vi "extractObjectPrivateDataValues.vi"(7 "error in (no error)":errorcluster, 8 "classPrivateDataDefaults":variant[](array[variant]), 9 "Object in":refnum<class>) -> (0 "error out":errorcluster, 2 "objectPrivateData":variant[](array[variant]))   [LabVIEW 2020, in "openg_variant.lvlib" / "Reflection.lvclass"]
doc: "Returns object Private Data values for the complete class hierarchy.\nClass Private Data defaults must be passed as an array of Variants where each element is a cluster of class private data with element 0 being the current class and the last element is the top ancestor class.\n\nGCraftsman JSON Object Serialization Toolkit\nwww.GCraftsman.com\nCopyright (c) 2017, GCraftsman"
uses:
  Reflection.lvclass
  Reflection.lvclass/Reflection.ctl
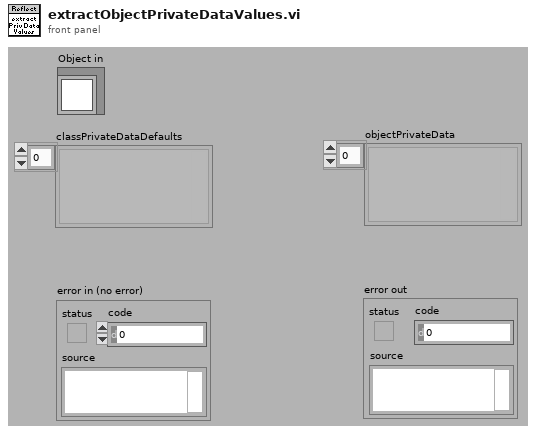
[diagram p1: front panel]
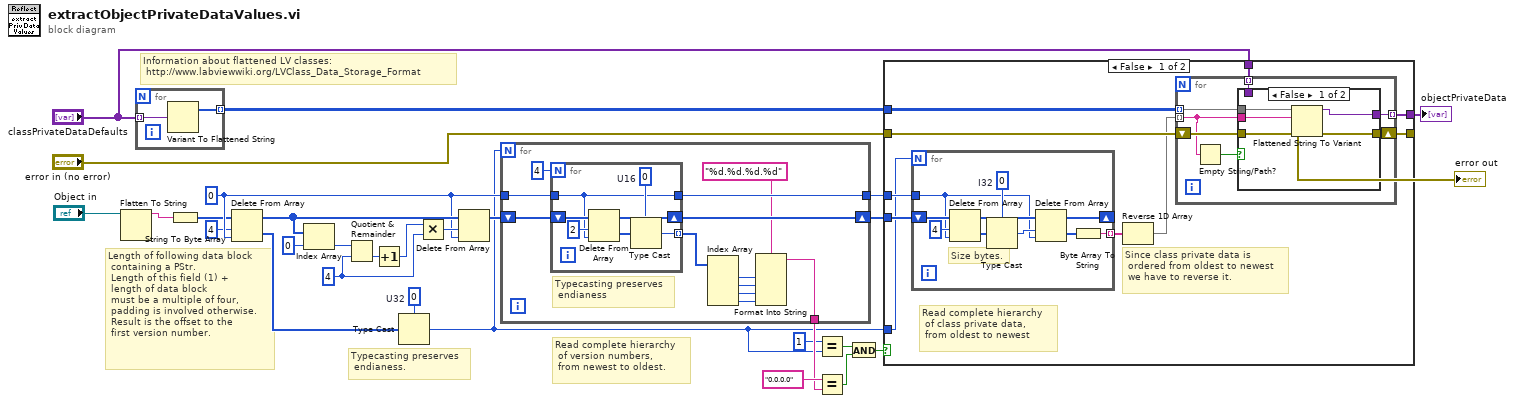
[diagram p0: block diagram]
diagram:
  w4 = u32 0  # U32
  w8 = u8 4 ("y")
  w19 = 0 ("index")
  # "Read complete hierarchy\n of version numbers,\n from newest to oldest."
  # "Information about flattened LV classes:\n http://www.labviewwiki.org/LVClass_Data_Storage_Format"
  # "Typecasting preserves\n endianess."
  # "Length of following data block\n containing a PStr.\n Length of this field (1) +\n length of data block\n must be a multiple of four,\n padding is involved otherwise.\n Result is the offset to the\n first version number."
  n1 = Flatten To String(anything="Object in") -> (data string=w1:string)  [unwired: 3 in, 2 out]
  n2 = for {
    tunnel: [w31] -> w14 mode=indexing
    tunnel: "classPrivateDataDefaults" -> [w30] mode=indexing
    n3 = Variant To Flattened String(Variant=w30) -> (1:w31:i16[])  [unwired: 1 out]
  }
  n4 = String To Byte Array(string=w1) -> (unsigned byte array=w16:u8[])
  n5 = Delete From Array(array=w16, length=4 ("offset (0)"), index=w19) -> (deleted portion=w6:u8[], array with subset deleted=w22:u8[])
  n6 = Index Array(array=w22, index=0) -> (element=w11:u8)
  n7 = Quotient & Remainder(x=w11, y=w8) -> (floor(x/y)=w10:u8)  [unwired: 1 out]
  n8 = Increment(x=w10) -> (x+1=w9:u8)
  n9 = Type Cast(type=w4, x=w6) -> (*(type *) &x=w5:u32)
  n10 = Multiply(x=w9, y=w8) -> (x*y=w21:u8)
  n11 = Delete From Array(array=w22, length=w21, index=w19) -> (array with subset deleted=w17:u8[])  [unwired: 1 out]
  n12 = for {
    N: w5 -> [_]
    shift-right: [w42] -> w18
    shift-left: w17 -> [w43]
    tunnel: w19 -> [w41]
    tunnel: [w39] -> w20
    tunnel: [w40] -> w24
    # "Typecasting preserves\n endianess"
    n13 = for {
      N: 4 -> [_]
      shift-right: [w48] -> w42
      shift-left: w43 -> [w50]
      tunnel: w41 -> [w44]
      tunnel: [w45] -> w36 mode=indexing
      tunnel: [w44] -> w39
      w46 = u16 0  # U16
      n14 = Delete From Array(array=w50, length=2, index=w44) -> (deleted portion=w47:u8[], array with subset deleted=w48:u8[])
      n15 = Type Cast(type=w46, x=w47) -> (*(type *) &x=w45:u16)
    }
    n16 = Index Array(array=w36) -> (element #1=w35:u16, element #2=w34:u16, element #3=w33:u16, element #4=w32:u16)  [unwired: 4 in]
    n17 = Format Into String(format string="%d.%d.%d.%d", w35, w34, w33, w32) -> (resulting string=w40:string)  [unwired: 2 in, 1 out]
  }
  n18 = Equal?(x=u32 1, y=w5) -> (x = y?=w26:bool)
  n19 = Equal?(x="0.0.0.0", y=w24) -> (x = y?=w27:bool)
  n20 = And(x=w26, y=w27) -> (x .and. y?=w28:bool)
  n21 = case shown="False" w28 {
    tunnel: w14 -> [w60 _]
    tunnel: [w55 w86] -> w29
    tunnel: w18 -> [w59 _]
    tunnel: w20 -> [w58 _]
    tunnel: w5 -> [w57 _]
    tunnel: [w56 w85] -> w13
    tunnel: "error in (no error)" -> [w54 w85]
    tunnel: "classPrivateDataDefaults" -> [w51 w86]
    frame False {
      # "Since class private data is\n ordered from oldest to newest\n we have to reverse it."
      # "Read complete hierarchy\n of class private data,\n from oldest to newest"
      n22 = for {
        N: w57 -> [_]
        shift-right: [w79] -> _
        shift-left: w59 -> [w84]
        tunnel: w58 -> [w77]
        tunnel: [w75] -> w53 mode=indexing
        w82 = 0  # I32
        # "Size bytes."
        n23 = Delete From Array(array=w84, length=4, index=w77) -> (deleted portion=w81:u8[], array with subset deleted=w80:u8[])
        n24 = Type Cast(type=w82, x=w81) -> (*(type *) &x=w78:i32)
        n25 = Delete From Array(array=w80, length=w78, index=w77) -> (deleted portion=w76:u8[], array with subset deleted=w79:u8[])
        n26 = Byte Array To String(unsigned byte array=w76) -> (string=w75:string)
      }
      n27 = Reverse 1D Array(array=w53) -> (reversed array=w52:string[])
      n28 = for {
        tunnel: w60 -> [w67] mode=indexing
        tunnel: [w64] -> w55 mode=indexing
        tunnel: w52 -> [w63] mode=indexing
        shift-right: [w65] -> w56
        shift-left: w54 -> [w66]
        tunnel: w51 -> [w61] mode=indexing
        n29 = Empty String/Path?(string/path=w63) -> (empty?=w62:bool)
        n30 = case shown="False" w62 {
          tunnel: w67 -> [w72 _]
          tunnel: w66 -> [w71 w73]
          tunnel: w63 -> [w70 _]
          tunnel: [w69 w73] -> w65
          tunnel: [w68 w74] -> w64
          tunnel: w61 -> [_ w74]
          frame False {
            n31 = Flattened String To Variant(4:w71, 6:w70, 7:w72) -> (0:w69:errorcluster, 3:w68:variant)
          }
          frame True {
            # "No data in this object.\nUse default value."
          }
        }
      }
    }
    frame True {
      # "// Version equals 0.0.0.0 and inheritance level is 1 (parent is LV object).\n// This means the private data cluster of the input object is empty.\n// Thus we return the default class private data"
    }
  }
  "objectPrivateData" <- w29
  "error out" <- w13
